vi "HFR500 Tx Rx.vi"(4 "String to Write":string="\u0002ÿSREM K0\u0003", 5 "TCP Network Connection in":refnum<k5>) -> (0 "error out":errorcluster, 2 "RX String (ASCII)":string)   [LabVIEW 2020]
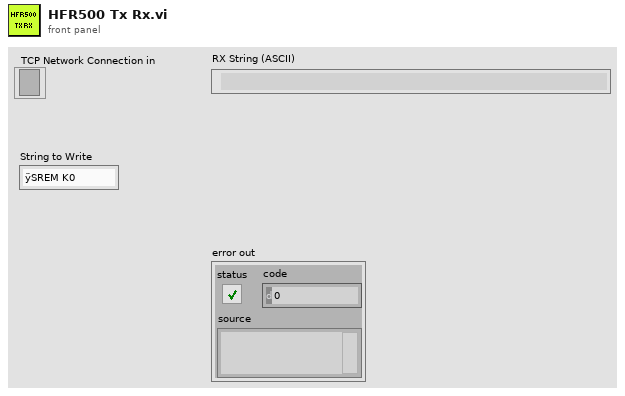
[diagram p1: front panel]
types:
  T1 = enum16{"Standard", "Buffered", "CRLF", "Immediate"}
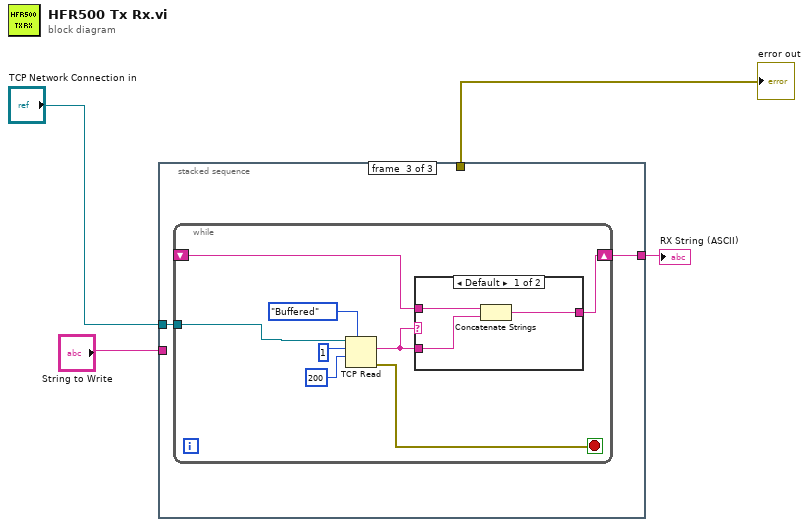
[diagram p0: block diagram]
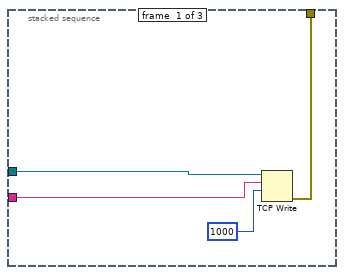
[diagram p2: hidden frame]
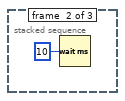
[diagram p3: hidden frame]
diagram:
  n1 = stacked-sequence {
    tunnel: "TCP Network Connection in" -> [w7 _ w11]
    tunnel: [w6 _ _] -> w2
    tunnel: "String to Write" -> [w5 _ _]
    tunnel: [_ _ w10] -> w3
    frame #0 {
      n2 = TCP Write(connection ID=w7, data in=w5, 9:1000 ("timeout ms (25000)")) -> (error out=w6:errorcluster)  [unwired: 1 in, 2 out]
    }
    frame #1 {
      n3 = Wait (ms)(milliseconds to wait=u32 10) -> ()  [unwired: 1 out]
    }
    frame #2 {
      n4 = while {
        tunnel: w11 -> [w14]
        shift-right: [w13] -> w10
        shift-left: _ -> [w12]
        stop <- w15 stop-if-true
        n5 = TCP Read(connection ID=w14, bytes to read=1, 7:T1."Buffered" ("mode (standard)"), 9:200 ("timeout ms (25000)")) -> (data out=w16:string, error out=w15:errorcluster)  [unwired: 1 in, 1 out]
        n6 = case shown="Default" w16 {
          tunnel: w12 -> [w21 _]
          tunnel: [w22 w23] -> w13
          tunnel: w16 -> [w20 w23]
          frame Default {
            n7 = Concatenate Strings(w21, w20) -> (w22:string)
          }
          frame "\u0002" {
            # "Start of string"
          }
        }
      }
    }
  }
  "RX String (ASCII)" <- w3
  "error out" <- w2
